vi "Main.vi"() -> ()   [LabVIEW 2013]
uses:
  Camera/lib/atmcd32d.llb/Shutter_type typedef.ctl
  Camera/lib/atmcd32d.llb/Shutter_mode typedef.ctl
  Utilities/controls/ctlSeqFNs_PI_SysNr.ctl
  Variables/StartStopMesaurement.vi
  Variables/GlobalExitVar.vi
  Variables/GlobalGetMesaurementStatus.vi
  Variables/GlobalSetGetConfigureCamera.vi
  Variables/ccdChipPixels.vi
  Variables/SavPath.vi
  Variables/GetPicture.vi
  Variables/StopGetPic.vi
  Variables/GlobalDevice.vi
  Variables/ScanrangeX.vi
  Variables/ScanrangeY.vi
  Variables/MesaurementModus.vi
  Variables/GlobalSetGetPixelOfRoi.vi
  Variables/GlobalSetConfigurationPhysikalInstruments.vi
  Variables/GlobalGetBeamDiagnostics.vi
  Variables/GlobalStopGetBeamDiagnostics.vi
panel:
  in  "Cams":enum32{"Acquisition", "Postprocessing"}(tab)
  out "Point":dbl[][](graph)
  out "Image Out":T1(plugin-control)
  in  "Gain::Value":dbl=16.0 min=16.0 max=64.0 step=1.0
  in  "Brightness::Value":dbl=127.0 min=0.0 max=254.0 step=1.0
  out "Image Number":u32
  out "Frame Rate":dbl
  in  "Stop Beam Diagnostic":bool
  in  "Get Beam Diagnostic":bool
  out "Final":dbl[][](graph)
  out "Confocal":dbl[][](graph)
  out "ISM":dbl[][](graph)
  in  "error in (no error)":errorcluster
  in  "Tab Control":enum32{"General"}(tab)
  in  "Check":bool
  in  "Stepsize Y":dbl format="%.2f"
  in  "Stepsize X":dbl format="%.2f"
  in  "Stepsize Z":dbl=10.0 format="%.2f"
  out "MesaurmentWarn":bool
  in  "Exposure (sec)":dbl=10.0 format="%.5f"
  in  "ModusMesaurement":enum32{"Fast", "Step"}(radio)
  in  "Scanrange Y":dbl format="%.2f"
  in  "Scanrange X":dbl format="%.2f"
  in  "Set Temp":bool
  in  "OpenShutter":bool
  in  "Emergency Exit":bool
  in  "Camera Settings":bool
  in  "GetPicture":bool
  in  "Stop Get Pic":bool
  in  "Close":bool
  in  "Start Measurement":bool
  in  "Move Mirror":bool
  in  "Move Scanner":bool
  in  "Set Workspace":bool
  in  "Laser Power":bool
  in  "AOTF Settings":bool
  in  "Device Choser":enum32{"Stage", "Mirror"}(radio)
  in  "Set CCD":bool
  in  "Startpoint X":dbl format="%.2f"
  in  "Startpoint Y":dbl format="%.2f"
  in  "Startpoint Z":dbl format="%.2f"
  in  "Scanrange Z":dbl=10.0 format="%.2f"
  in  "WAV":bool
  out "Writing":bool
  # "Data From Andor Camera Piped From Aquisition Process"
  # "Beam Diagnostic Camera"
  # "Beam Diagnostic Camera Controll"
  # "Define Where To Save the Mesaurement Data"
  # "Navigate In Sample Space & Choose Kinetic Device"
  # "Laser & AOTF/AOM"
  # "Data Acquisition Camera"
  # "Preview"
  # "Mesaurement Processs"
  # "Controlled & Emergency Shutdown"
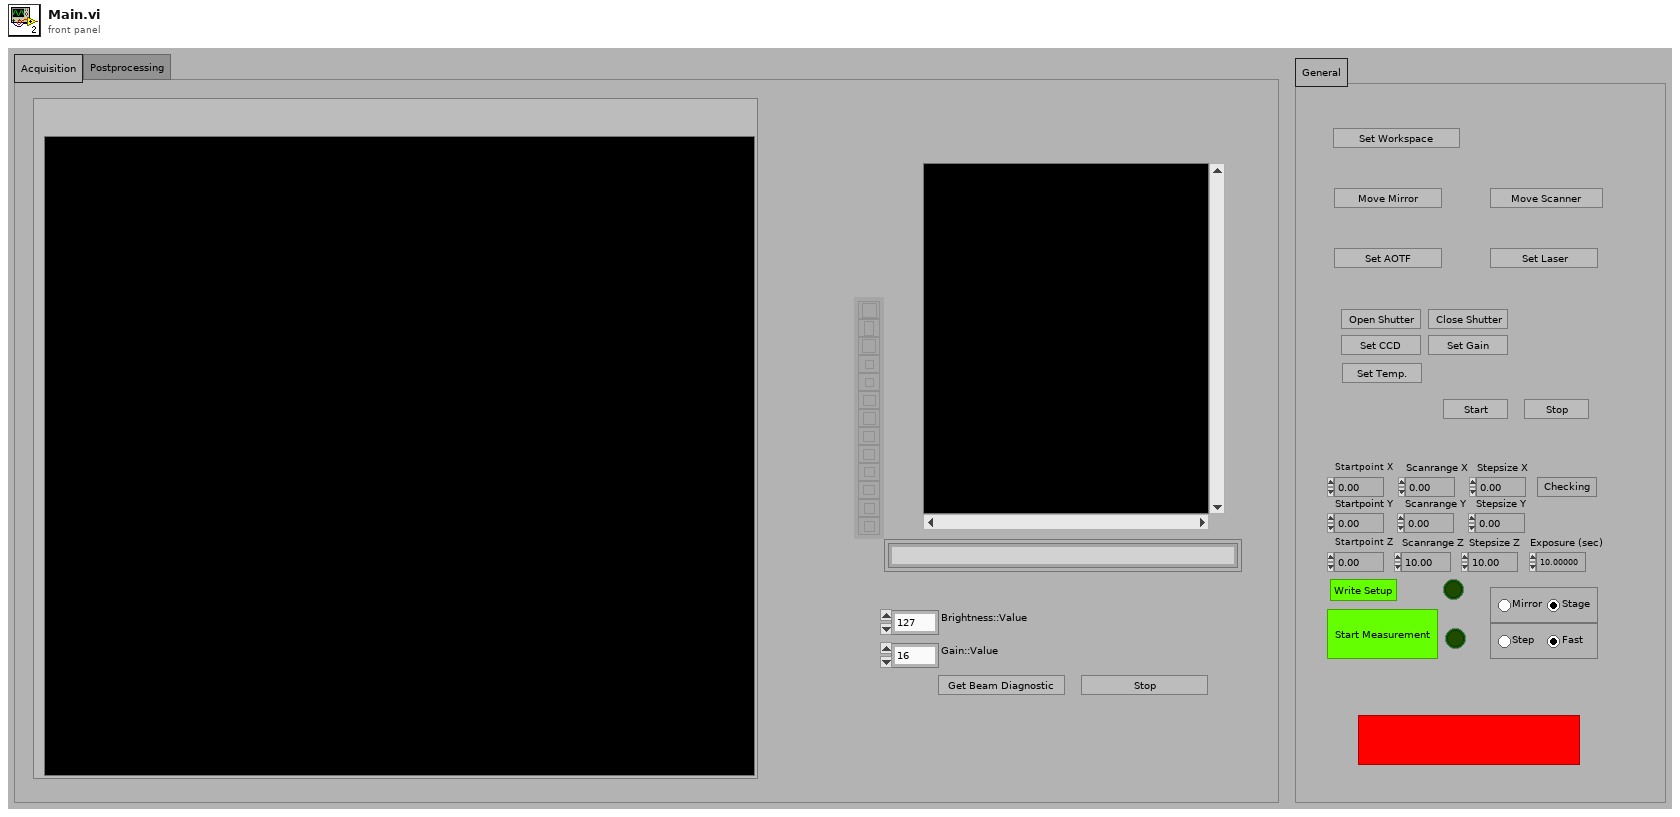
[diagram p1: front panel]
types:
  T1 = typedef "IMAQ Image.ctl" = refnum<image>
  T2 = typedef "Shutter_type typedef.ctl" = enum16{"TTL Low", "TTL High"}
  T3 = typedef "Shutter_mode typedef.ctl" = enum16{"Auto", "Open", "Close"}
  T4 = typedef "ctlSeqFNs_PI_SysNr.ctl" = enum16{"Zero", "E517", "E710"}
  T5 = cluster{"Conn. Axes scanner[0]":string, "Conn. Axes scanner[1]":string, "Conn. Axes scanner[2]":string}
  T6 = cluster{"Points":dbl, "J":dbl, "X length ":dbl, "J":dbl}
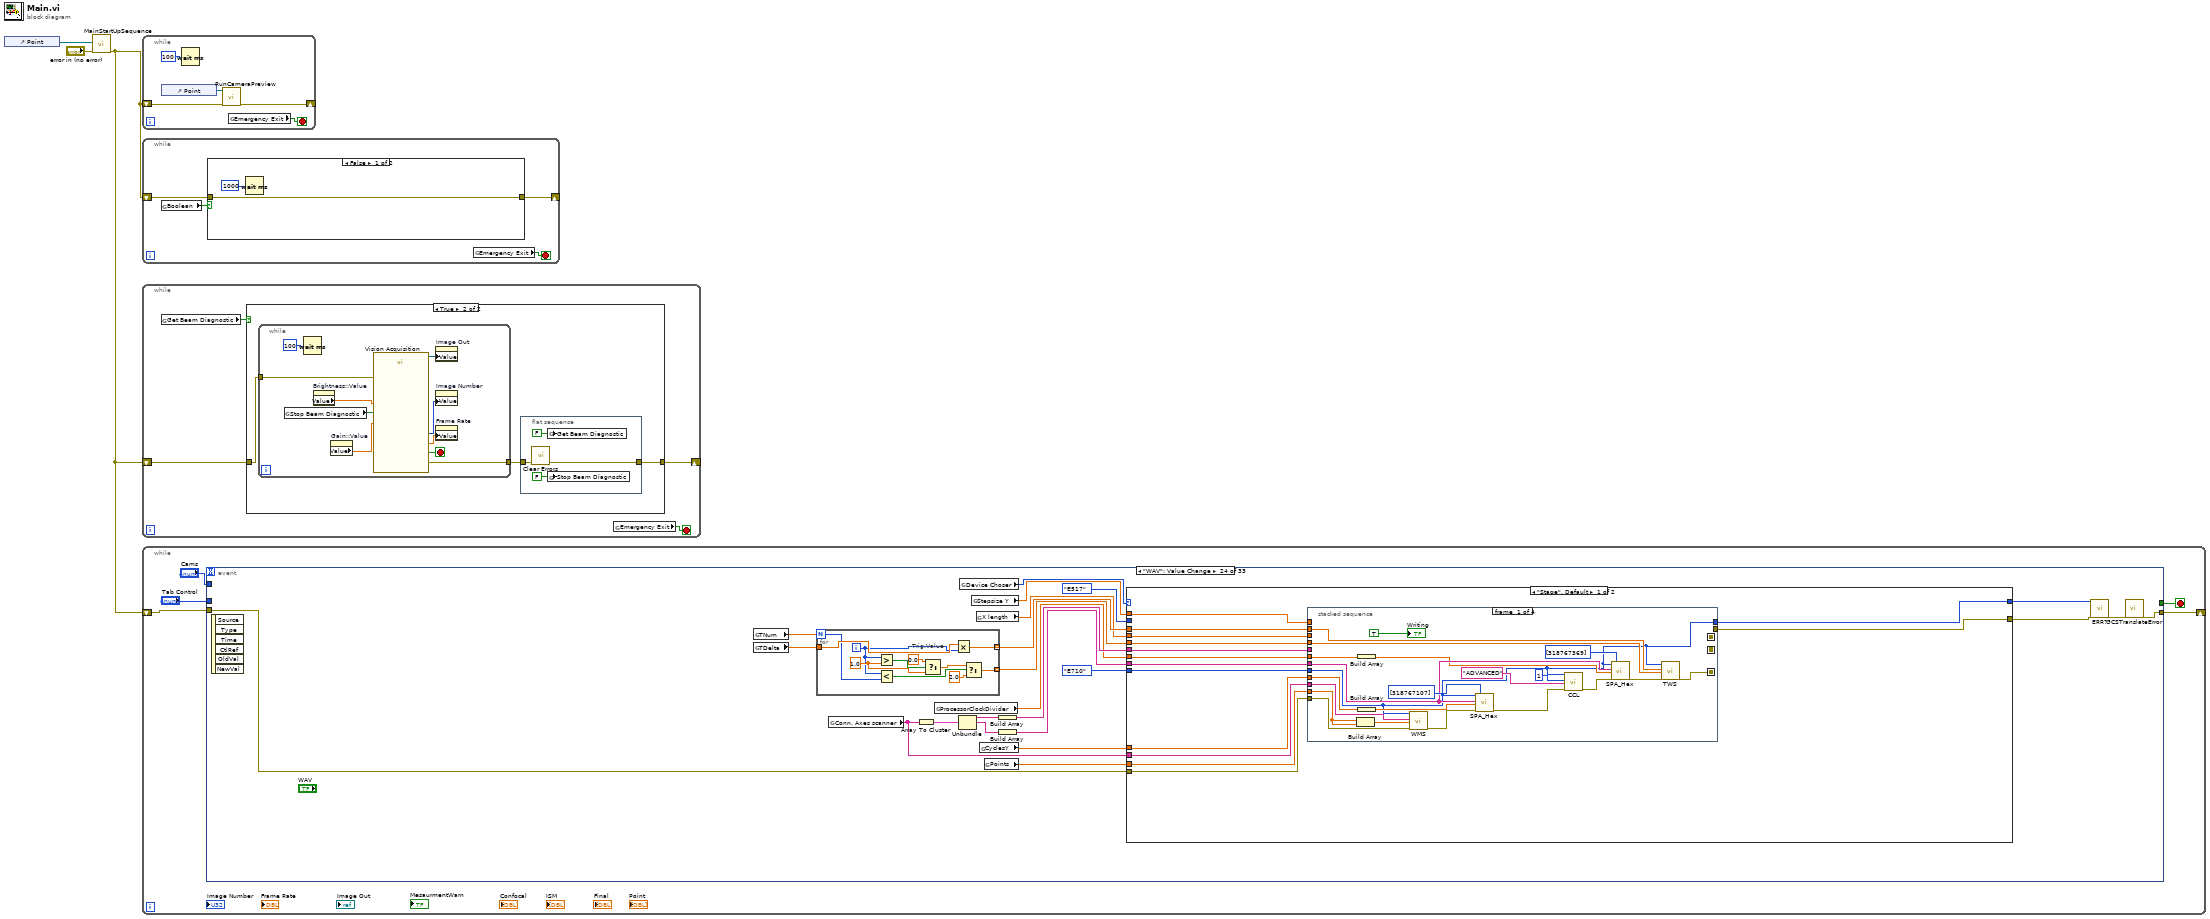
[diagram p0: block diagram]
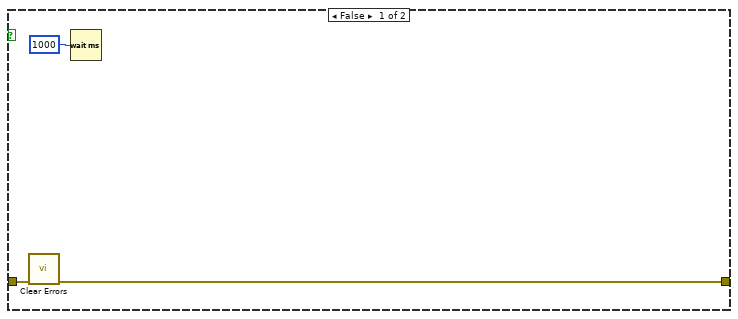
[diagram p2: hidden frame]
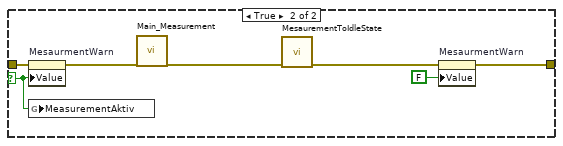
[diagram p3: hidden frame]
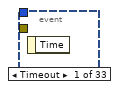
[diagram p4: hidden frame]
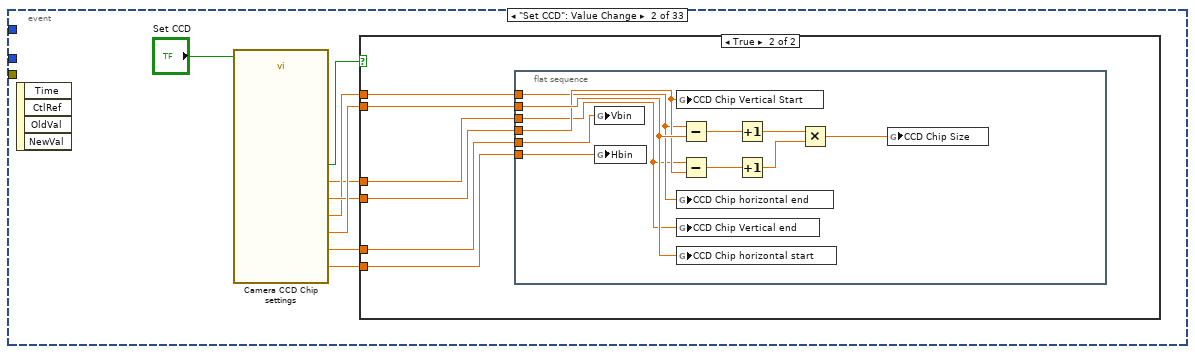
[diagram p5: hidden frame]
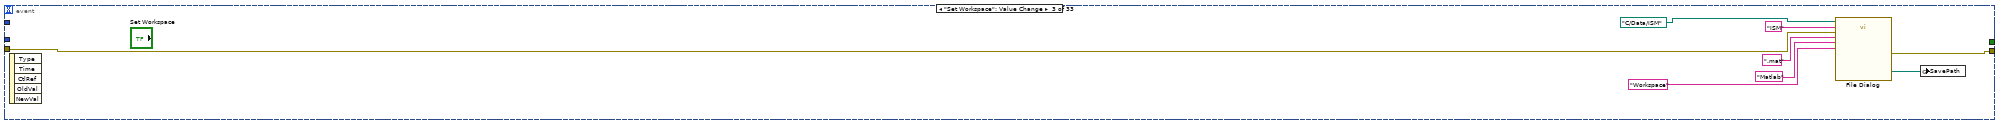
[diagram p7: hidden frame]
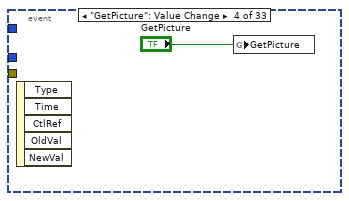
[diagram p8: hidden frame]
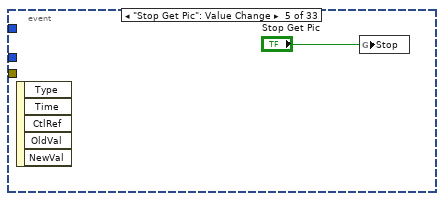
[diagram p9: hidden frame]
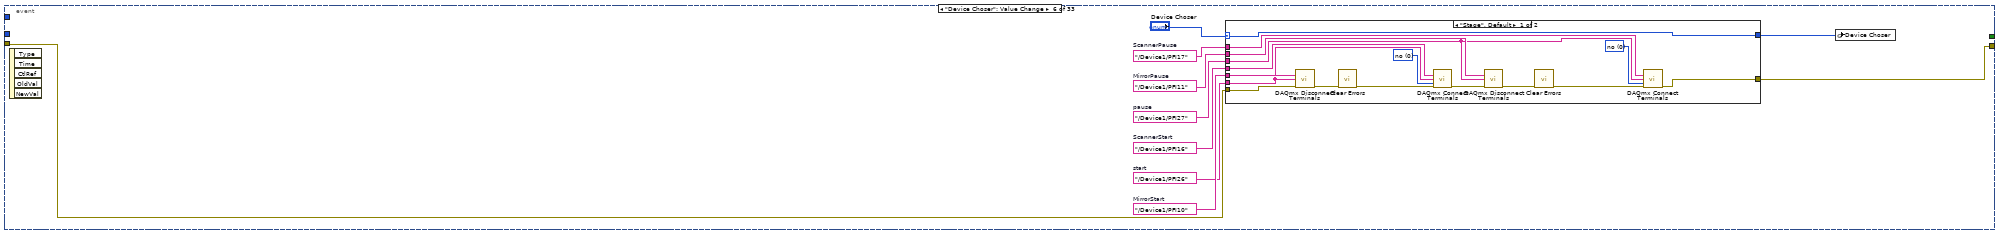
[diagram p10: hidden frame]
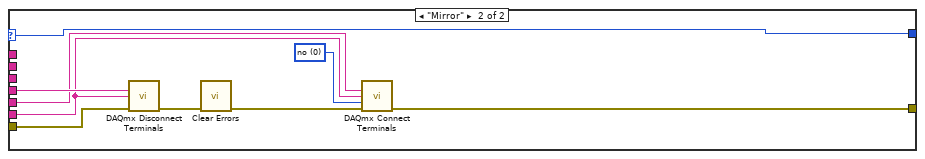
[diagram p11: hidden frame]
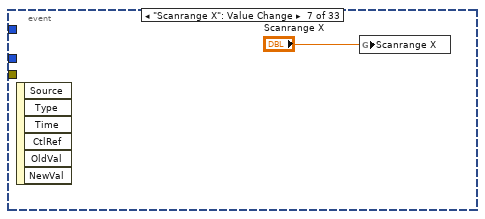
[diagram p12: hidden frame]
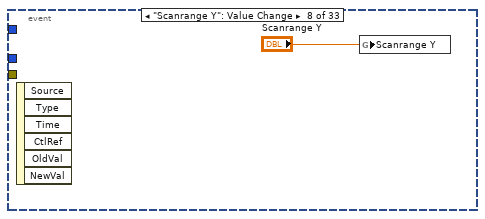
[diagram p13: hidden frame]
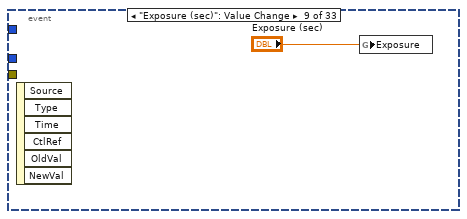
[diagram p14: hidden frame]
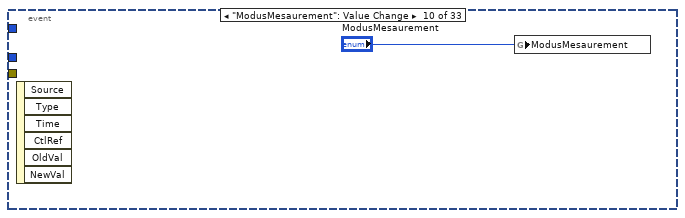
[diagram p15: hidden frame]
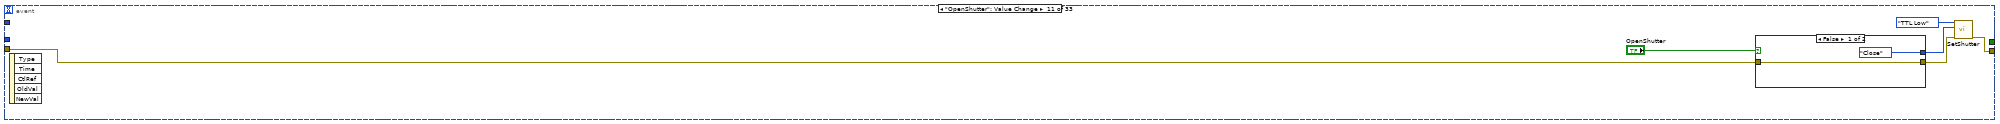
[diagram p16: hidden frame]
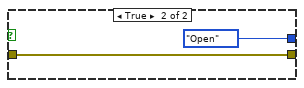
[diagram p17: hidden frame]
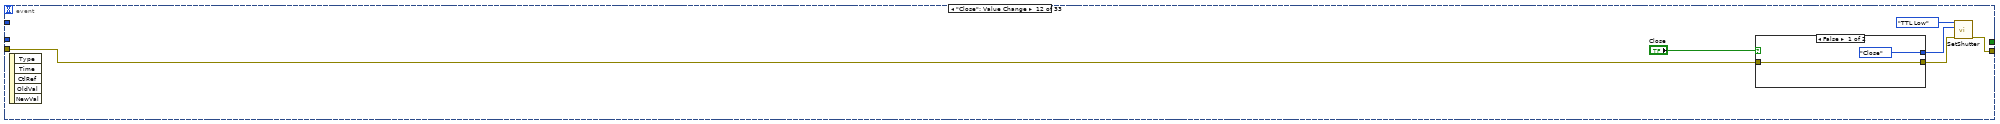
[diagram p18: hidden frame]
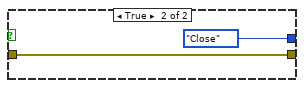
[diagram p19: hidden frame]
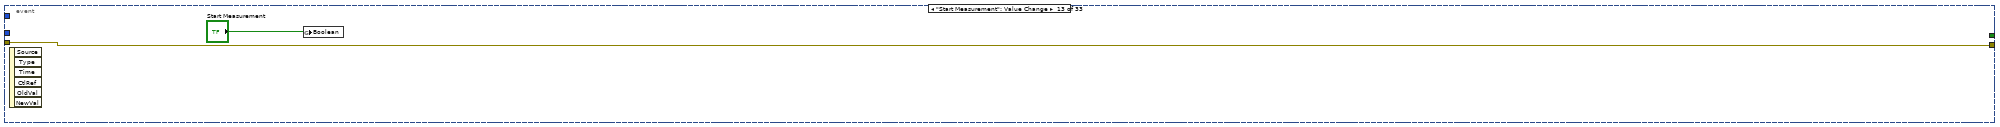
[diagram p20: hidden frame]
diagram:
  n1 = control-ref of="Point"() -> (w1:refnum<vi>)
  n2 = call "MainStartUpSequence.vi"("IntGraph Refnum"=w1, "error in (no error)"="error in (no error)") -> ("error out"=w2:errorcluster)  [unwired: 15 in, 2 out]
  n3 = while {
    shift-right: [w6] -> _
    shift-left: w2 -> [w7]
    stop <- w8 stop-if-true
    n4 = control-ref of="Point"() -> (w5:refnum<vi>)
    n5 = Wait (ms)(milliseconds to wait=u32 100) -> ()  [unwired: 1 out]
    n6 = call "RunCameraPreview.vi"("error in (no error)"=w7, "IntensityGraph in"=w5) -> ("error out"=w6:errorcluster)  [unwired: 9 in]
    n7 = global read "GlobalExitVar.vi" "Emergency Exit"() -> (w8:bool)
  }
  n8 = while {
    shift-right: [w11] -> _
    shift-left: w2 -> [w12]
    stop <- w9 stop-if-true
    n9 = global read "StartStopMesaurement.vi" "Boolean"() -> (w10:bool)
    n10 = case shown="False" w10 {
      selector: w10 -> [_ w15]
      tunnel: w12 -> [w13 w17]
      tunnel: [w13 w19] -> w11
      frame False {
        n11 = Wait (ms)(milliseconds to wait=u32 1000) -> ()  [unwired: 1 out]
      }
      frame True {
        n12 = property on="MesaurmentWarn" class="Bool (strict)"(error in=w17, "Value"=w15) -> (error out=w16:errorcluster)  [unwired: 1 in, 1 out]
        n13 = global write "GlobalGetMesaurementStatus.vi" "MeasurementAktiv"(w15) -> ()
        n14 = call "Main_Measurement.vi"("error in"=w16) -> ("error out"=w21:errorcluster)  [unwired: 18 in]
        n15 = call "MesaurementToIdleState.vi"("error in (no error)"=w21) -> ("error out"=w20:errorcluster)  [unwired: 10 in]
        n16 = property on="MesaurmentWarn" class="Bool (strict)"(error in=w20, "Value"=FALSE ("MesaurmentWarn")) -> (error out=w19:errorcluster)  [unwired: 1 in, 1 out]
      }
    }
    n17 = global read "GlobalExitVar.vi" "Emergency Exit"() -> (w9:bool)
  }
  n18 = while {
    shift-right: [w23] -> _
    shift-left: w2 -> [w24]
    stop <- w25 stop-if-true
    n19 = global read "GlobalGetBeamDiagnostics.vi" "Get Beam Diagnostic"() -> (w22:bool)
    n20 = case shown="True" w22 {
      tunnel: w24 -> [w27 w31]
      tunnel: [w26 w30] -> w23
      frame False {
        n21 = call <vilib>:"Clear Errors.vi"("error in (no error)"=w27) -> ("error out"=w26:errorcluster)  [unwired: 6 in]
        n22 = Wait (ms)(milliseconds to wait=u32 1000) -> ()  [unwired: 1 out]
      }
      frame True {
        n23 = while {
          tunnel: w31 -> [w40]
          tunnel: [w39] -> w29
          stop <- w41 stop-if-true
          n24 = global read "GlobalStopGetBeamDiagnostics.vi" "Stop Beam Diagnostic"() -> (w38:bool)
          n25 = Wait (ms)(milliseconds to wait=u32 100) -> ()  [unwired: 1 out]
          n26 = property on="Brightness::Value" class="DigNum (strict)"() -> ("Value"=w37:dbl)  [unwired: 2 in, 2 out]
          n27 = property on="Gain::Value" class="DigNum (strict)"() -> ("Value"=w36:dbl)  [unwired: 2 in, 2 out]
          n28 = call "Vision Acquisition"("Brightness::Value"=w37, "Stop (F)"=w38, "Gain::Value"=w36, "error in"=w40) -> ("Image Out"=w33:T1, "Image Number"=w35:u32, "Frame Rate"=w34:dbl, "Stopped"=w41:bool, "error out"=w39:errorcluster)  [unwired: 19 in]
          n29 = property on="Image Out" class="ImageControl"("Value"=w33) -> ()  [unwired: 2 in, 2 out]
          n30 = property on="Image Number" class="DigNum (strict)"("Value"=w35) -> ()  [unwired: 2 in, 2 out]
          n31 = property on="Frame Rate" class="DigNum (strict)"("Value"=w34) -> ()  [unwired: 2 in, 2 out]
        }
        n32 = flat-sequence {
          tunnel: [w42] -> w30
          tunnel: w29 -> [w43]
          frame #0 {
            n33 = call <vilib>:"Clear Errors.vi"("error in (no error)"=w43) -> ("error out"=w42:errorcluster)  [unwired: 6 in]
            n34 = global write "GlobalGetBeamDiagnostics.vi" "Get Beam Diagnostic"(FALSE ("Get Beam Diagnostic")) -> ()
            n35 = global write "GlobalStopGetBeamDiagnostics.vi" "Stop Beam Diagnostic"(FALSE ("Stop Beam Diagnostic")) -> ()
          }
        }
      }
    }
    n36 = global read "GlobalExitVar.vi" "Emergency Exit"() -> (w25:bool)
  }
  n37 = while "User Events" {
    shift-right: [w48] -> _
    shift-left: w2 -> [w50]
    stop <- w49 stop-if-true
    n38 = event shown="[23] \"WAV\": Value Change" {
      selector: _ -> [_ _ _ _ _ _ _ _ _ _ _ _ _ _ _ _ _ _ _ _ _ _ _ _ _ _ _ _ _ _ _ _ _]
      dyn-events: _ -> [_ _ _ _ _ _ _ _ _ _ _ _ _ _ _ _ _ _ _ _ _ _ _ _ _ _ _ _ _ _ _ _ _]
      timeout: _ -> [_ _ _ _ _ _ _ _ _ _ _ _ _ _ _ _ _ _ _ _ _ _ _ _ _ _ _ _ _ _ _ _ _]
      tunnel: [_ _ w77 _ _ w90 _ _ _ _ w126 w136 w146 w148 w161 w179 _ _ _ _ _ _ _ w281 _ w431 _ _ w495 w496 _ _ w502] -> w48
      tunnel: w50 -> [_ _ w76 _ _ w91 _ _ _ _ w128 w138 w146 w153 w165 w183 _ _ _ _ _ _ _ w276 w400 w422 _ _ w494 w497 _ _ w506]
      tunnel: [_ _ _ _ _ _ _ _ _ _ _ _ _ _ _ _ _ _ _ _ _ _ _ _ _ _ _ _ _ _ _ _ w501] -> w49
      tunnel: "Tab Control" -> [_ _ _ _ _ _ _ _ _ _ _ _ _ _ _ _ _ _ _ _ _ _ _ _ _ _ _ _ _ _ _ _ _]
      tunnel: "Cams" -> [_ _ _ _ _ _ _ _ _ _ _ _ _ _ _ _ _ _ _ _ _ _ _ _ _ _ _ _ _ _ _ _ _]
      event Timeout {
        n39 = event-data() -> ()  [unwired: 1 in, 1 out]
      }
      event "Set CCD": Value Change {
        n40 = event-data() -> ()  [unwired: 1 in, 4 out]
        n41 = call "Camera CCD Chip settings"("Enable"="Set CCD") -> ("Horizontal Binning"=w51:dbl, "Vertical Binning"=w56:dbl, "CCD Chip Horizontal Start"=w55:dbl, "CCD Chip Horizontal End"=w53:dbl, "CCD Chip Vertical Start"=w54:dbl, "CCD Chip Vertical End"=w52:dbl, "OK"=w57:bool)  [unwired: 11 in, 1 out]
        n42 = case shown="True" w57 {
          tunnel: w56 -> [_ w64]
          tunnel: w55 -> [_ w63]
          tunnel: w54 -> [_ w62]
          tunnel: w53 -> [_ w61]
          tunnel: w52 -> [_ w60]
          tunnel: w51 -> [_ w59]
          frame False {
          }
          frame True {
            n43 = flat-sequence {
              tunnel: w64 -> [w70]
              tunnel: w63 -> [w69]
              tunnel: w62 -> [w68]
              tunnel: w61 -> [w67]
              tunnel: w60 -> [w66]
              tunnel: w59 -> [w65]
              frame #0 {
                n44 = global write "GlobalSetGetConfigureCamera.vi" "Vbin"(w70) -> ()
                n45 = global write "GlobalSetGetConfigureCamera.vi" "Hbin"(w65) -> ()
                n46 = global write "ccdChipPixels.vi" "CCD Chip Vertical Start"(w68) -> ()
                n47 = global write "ccdChipPixels.vi" "CCD Chip horizontal end"(w67) -> ()
                n48 = global write "ccdChipPixels.vi" "CCD Chip Vertical end"(w66) -> ()
                n49 = global write "ccdChipPixels.vi" "CCD Chip horizontal start"(w69) -> ()
                n50 = Subtract(x=w67, y=w69) -> (x-y=w72:dbl)
                n51 = Subtract(x=w66, y=w68) -> (x-y=w71:dbl)
                n52 = Increment(x=w72) -> (x+1=w74:dbl)
                n53 = Increment(x=w71) -> (x+1=w73:dbl)
                n54 = Multiply(x=w74, y=w73) -> (x*y=w75:dbl)
                n55 = global write "ccdChipPixels.vi" "CCD Chip Size"(w75) -> ()
              }
            }
          }
        }
      }
      event "Set Workspace": Value Change {
        n56 = event-data() -> ()  [unwired: 1 in, 5 out]
        n57 = call "File Dialog"("start path"=path "C:/Data/ISM", "button label"="Workspace", "default name"="ISM", "error in"=w76, "pattern (all files)"=".mat", "pattern label"="Matlab") -> ("selected path"=w82:path, "error out"=w77:errorcluster)  [unwired: 6 in, 2 out]
        n58 = global write "SavPath.vi" "SavePath"(w82) -> ()
      }
      event "GetPicture": Value Change {
        n59 = event-data() -> ()  [unwired: 1 in, 5 out]
        n60 = global write "GetPicture.vi" "GetPicture"("GetPicture") -> ()
      }
      event "Stop Get Pic": Value Change {
        n61 = event-data() -> ()  [unwired: 1 in, 5 out]
        n62 = global write "StopGetPic.vi" "Stop"("Stop Get Pic") -> ()
      }
      event "Device Choser": Value Change {
        w87 = tag "/Device1/PFI17"  # ScannerPause
        w88 = tag "/Device1/PFI11"  # MirrorPause
        w86 = tag "/Device1/PFI26"  # start
        w89 = tag "/Device1/PFI27"  # pause
        w95 = tag "/Device1/PFI16"  # ScannerStart
        w94 = tag "/Device1/PFI10"  # MirrorStart
        n63 = event-data() -> ()  [unwired: 1 in, 5 out]
        n64 = case shown="\"Stage\", Default" "Device Choser" {
          selector: "Device Choser" -> [w104 w112]
          tunnel: w91 -> [w110 w118]
          tunnel: [w96 w120] -> w90
          tunnel: w94 -> [w108 w113]
          tunnel: w86 -> [w107 w116]
          tunnel: w95 -> [w109 w117]
          tunnel: [w104 w112] -> w92
          tunnel: w89 -> [w98 _]
          tunnel: w88 -> [w100 _]
          tunnel: w87 -> [w99 _]
          frame "Stage", Default {
            w103 = 0 items=["no", "yes"] ("invert polarity")
            w111 = 0 items=["no", "yes"] ("invert polarity")
            n65 = call <vilib>:"DAQmx Disconnect Terminals.vi"("source terminal"=w108, "destination terminal"=w107, "error in"=w110) -> ("error out"=w106:errorcluster)  [unwired: 12 in]
            n66 = call <vilib>:"Clear Errors.vi"("error in (no error)"=w106) -> ("error out"=w105:errorcluster)  [unwired: 6 in]
            n67 = call <vilib>:"DAQmx Connect Terminals.vi"("source terminal"=w109, "destination terminal"=w107, "invert polarity"=w111, "error in"=w105) -> ("error out"=w97:errorcluster)  [unwired: 11 in]
            n68 = call <vilib>:"DAQmx Disconnect Terminals.vi"("source terminal"=w100, "destination terminal"=w98, "error in"=w97) -> ("error out"=w102:errorcluster)  [unwired: 12 in]
            n69 = call <vilib>:"Clear Errors.vi"("error in (no error)"=w102) -> ("error out"=w101:errorcluster)  [unwired: 6 in]
            n70 = call <vilib>:"DAQmx Connect Terminals.vi"("source terminal"=w99, "destination terminal"=w98, "invert polarity"=w103, "error in"=w101) -> ("error out"=w96:errorcluster)  [unwired: 11 in]
          }
          frame "Mirror" {
            w119 = 0 items=["no", "yes"] ("invert polarity")
            n71 = call <vilib>:"DAQmx Disconnect Terminals.vi"("source terminal"=w117, "destination terminal"=w116, "error in"=w118) -> ("error out"=w115:errorcluster)  [unwired: 12 in]
            n72 = call <vilib>:"Clear Errors.vi"("error in (no error)"=w115) -> ("error out"=w114:errorcluster)  [unwired: 6 in]
            n73 = call <vilib>:"DAQmx Connect Terminals.vi"("source terminal"=w113, "destination terminal"=w116, "invert polarity"=w119, "error in"=w114) -> ("error out"=w120:errorcluster)  [unwired: 11 in]
          }
        }
        n74 = global write "GlobalDevice.vi" "Device Choser"(w92) -> ()
      }
      event "Scanrange X": Value Change {
        n75 = event-data() -> ()  [unwired: 1 in, 6 out]
        n76 = global write "ScanrangeX.vi" "Scanrange X"("Scanrange X") -> ()
      }
      event "Scanrange Y": Value Change {
        n77 = event-data() -> ()  [unwired: 1 in, 6 out]
        n78 = global write "ScanrangeY.vi" "Scanrange Y"("Scanrange Y") -> ()
      }
      event "Exposure (sec)": Value Change {
        n79 = event-data() -> ()  [unwired: 1 in, 6 out]
        n80 = global write "GlobalSetGetConfigureCamera.vi" "Exposure"("Exposure (sec)") -> ()
      }
      event "ModusMesaurement": Value Change {
        n81 = event-data() -> ()  [unwired: 1 in, 6 out]
        n82 = global write "MesaurementModus.vi" "ModusMesaurement"("ModusMesaurement") -> ()
      }
      event "OpenShutter": Value Change {
        n83 = event-data() -> ()  [unwired: 1 in, 5 out]
        n84 = case shown="False" "OpenShutter" {
          tunnel: [Shutter_mode_typedef."Close" ("mode") Shutter_mode_typedef."Open" ("mode")] -> w130
          tunnel: w128 -> [w132 w133]
          tunnel: [w132 w133] -> w127
          frame False {
          }
          frame True {
          }
        }
        n85 = call "SetShutter.vi"("type"=Shutter_type_typedef."TTL Low", "mode"=w130, "error in (no error)"=w127) -> ("error out"=w126:errorcluster)  [unwired: 11 in, 1 out]
      }
      event "Close": Value Change {
        n86 = event-data() -> ()  [unwired: 1 in, 5 out]
        n87 = case shown="False" "Close" {
          tunnel: w138 -> [w141 w144]
          tunnel: [w141 w144] -> w137
          tunnel: [Shutter_mode_typedef."Close" ("mode") Shutter_mode_typedef."Close" ("mode")] -> w135
          frame False {
          }
          frame True {
          }
        }
        n88 = call "SetShutter.vi"("type"=Shutter_type_typedef."TTL Low", "mode"=w135, "error in (no error)"=w137) -> ("error out"=w136:errorcluster)  [unwired: 11 in, 1 out]
      }
      event "Start Measurement": Value Change {
        n89 = event-data() -> ()  [unwired: 1 in, 6 out]
        n90 = global write "StartStopMesaurement.vi" "Boolean"("Start Measurement") -> ()
      }
      event "Move Scanner": Value Change {
        n91 = event-data() -> ()  [unwired: 1 in, 6 out]
        n92 = call "Scanner kinetics"("error in (no error)"=w153) -> ("Go to Z-position"=w150:dbl, "Go to Y-position"=w151:dbl, "Go to X-position"=w152:dbl, "OK"=w149:bool, "error out"=w147:errorcluster)  [unwired: 14 in]
        n93 = case shown="True" w149 {
          tunnel: w152 -> [_ w159]
          tunnel: w151 -> [_ w158]
          tunnel: w150 -> [_ w157]
          tunnel: [w154 w156] -> w148
          tunnel: w147 -> [w154 w155]
          frame False {
          }
          frame True {
            n94 = call "Scanner_Mirror_configuration.vi"("POS X"=w159, "POS Y"=w158, "POS Z"=w157, "error in"=w155) -> ("error out"=w156:errorcluster)  [unwired: 15 in]
          }
        }
      }
      event "Move Mirror": Value Change {
        n95 = event-data() -> ()  [unwired: 1 in, 6 out]
        n96 = call "Mirror kinetics"("error in (no error)"=w165) -> ("Go to X-position"=w163:dbl, "Go to Y-position"=w164:dbl, "OK"=w160:bool, "error out"=w162:errorcluster)  [unwired: 15 in]
        n97 = case shown="True" w160 {
          tunnel: w164 -> [_ w170]
          tunnel: w163 -> [_ w169]
          tunnel: w162 -> [w166 w168]
          tunnel: [w166 w167] -> w161
          frame False {
          }
          frame True {
            n98 = call "MoveMirror.vi"("error in 2"=w168, "POS X rad"=w169, "POS Y rad"=w170) -> ("error out 2"=w167:errorcluster)  [unwired: 1 in]
          }
        }
      }
      event "Check": Value Change {
        n99 = event-data() -> ()  [unwired: 1 in, 6 out]
        n100 = global read "ScanrangeX.vi" "Scanrange X"() -> (w178:dbl)
        n101 = global read "ScanrangeY.vi" "Scanrange Y"() -> (w177:dbl)
        n102 = global read "GlobalSetGetPixelOfRoi.vi" "Stepsize Y"() -> (w188:dbl)
        n103 = global read "GlobalSetGetPixelOfRoi.vi" "Stepsize X"() -> (w191:dbl)
        n104 = global write "GlobalSetGetPixelOfRoi.vi" "X length"(w178) -> ()
        n105 = global write "GlobalSetGetPixelOfRoi.vi" "Y length"(w177) -> ()
        n106 = Quotient & Remainder(x=w178, y=w191) -> (x-y*floor(x/y)=w190:dbl)  [unwired: 1 out]
        n107 = Quotient & Remainder(x=w177, y=w188) -> (x-y*floor(x/y)=w189:dbl)  [unwired: 1 out]
        n108 = Greater Than 0?(x=w190) -> (x > 0?=w187:bool)
        n109 = Greater Than 0?(x=w189) -> (x > 0?=w186:bool)
        n110 = Or(x=w187, y=w186) -> (x .or. y?=w185:bool)
        n111 = case shown="True" w185 {
          tunnel: w183 -> [w232 w234]
          tunnel: [w232 w233] -> w180
          frame False {
          }
          frame True {
            n112 = call "Display Message to User3"("error in (no error)"=w234) -> ("error out"=w233:errorcluster)  [unwired: 9 in, 1 out]
          }
        }
        n113 = global read "GlobalSetGetConfigureCamera.vi" "Exposure"() -> (w171:sgl)
        n114 = global read "GlobalDevice.vi" "Device Choser"() -> (w198:enum32{"Stage", "Mirror"})
        n115 = global read "GlobalSetGetPixelOfRoi.vi" "Stack length"() -> (w192:dbl)
        n116 = case shown="\"Stage\", Default" w198 {
          tunnel: [w244 w255] -> w211
          tunnel: [w239 w251] -> w194
          tunnel: [w245 w256] -> w204
          tunnel: [w241 w250] -> w199
          tunnel: [w243 w254] -> w197
          tunnel: w178 -> [w245 w256]
          tunnel: w177 -> [w244 w255]
          tunnel: w188 -> [w243 w254]
          tunnel: w191 -> [w241 w250]
          tunnel: w171 -> [w240 w249]
          tunnel: [w238 w253] -> w193
          tunnel: w192 -> [w238 w253]
          tunnel: [w237 w248] -> w181
          tunnel: w180 -> [w237 w248]
          tunnel: [5000.0 ("input variable") 25000.0 ("input variable")] -> w173
          tunnel: [63488.0 ("input variable") 63488.0 ("input variable")] -> w174
          frame "Stage", Default {
            n117 = Divide(x=w241, y=w240) -> (x/y=w242:dbl)
            n118 = Round To Nearest(number=w242) -> (nearest integer value=w239:dbl)
          }
          frame "Mirror" {
            # "1 durch25000 fehlt speed calc \nbei spiegel anpassen dh 8.2.14"
            n119 = Divide(x=w250, y=w249) -> (x/y=w252:dbl)
            n120 = Round To Nearest(number=w252) -> (nearest integer value=w251:dbl)
          }
        }
        n121 = global read "GlobalSetGetPixelOfRoi.vi" "Stepsize Z"() -> (w196:dbl)
        n122 = while {
          tunnel: w211 -> [w231]
          tunnel: [w219] -> w210
          tunnel: [w230] -> w209
          tunnel: [w229] -> w208
          tunnel: [w228] -> w207
          tunnel: w204 -> [w227]
          tunnel: w199 -> [w226]
          tunnel: w197 -> [w225]
          tunnel: w196 -> [w224]
          tunnel: w194 -> [w218]
          tunnel: w193 -> [w223]
          tunnel: [w222] -> w184
          tunnel: [w221] -> w176
          tunnel: w174 -> [w220]
          shift-right: [w215] -> _
          shift-left: _ -> [w216]
          tunnel: w173 -> [w214]
          tunnel: [w213] -> w172
          i -> [w213]
          stop <- w217 stop-if-true
          n123 = formula code="CyclesY = floor (RangeY/StepY) + 1;\nCyclesZ = floor (RangeZ/StepZ) + 1;\nVmin = Clock/Memory * RangeX * (1 + CyclesY);\nPointsX = RangeX / Speed * 10000;\nTDelta = PointsX / RangeX * Trigger;\nTNum = floor ( PointsX / TDelta);"("RangeX"=w227, "RangeY"=w231, "RangeZ"=w223, "StepY"=w225, "StepZ"=w224, "Speed"=w218, "Trigger"=w226, "Clock"=w216, "Memory"=w220) -> ("Vmin"=w219:dbl, "CyclesY"=w221:dbl, "CyclesZ"=w228:dbl, "PointsX"=w222:dbl, "TDelta"=w230:dbl, "TNum"=w229:dbl)
          n124 = Greater?(x=w218, y=w219) -> (0:w217:bool)
          n125 = Divide(x=w214, y=w213) -> (x/y=w215:dbl)
        }
        n126 = global write "GlobalSetGetPixelOfRoi.vi" "Stepsize Y"(w197) -> ()
        n127 = global write "GlobalSetGetPixelOfRoi.vi" "Points"(w184) -> ()
        n128 = global write "GlobalSetGetPixelOfRoi.vi" "TDelta"(w209) -> ()
        n129 = global write "GlobalDevice.vi" "ProcessorClockDivider"(w172) -> ()
        n130 = global write "GlobalSetGetPixelOfRoi.vi" "TNum"(w208) -> ()
        n131 = global write "GlobalSetGetPixelOfRoi.vi" "CyclesY"(w176) -> ()
        n132 = global write "GlobalSetGetPixelOfRoi.vi" "CyclesZ"(w207) -> ()
        n133 = Less?(x=w194, y=w210) -> (x < y?=w212:bool)
        n134 = Divide(x=w204, y=w199) -> (x/y=w175:dbl)
        n135 = Subtract(x=w176, y=1.0) -> (x-y=w200:dbl)
        n136 = Multiply(x=w200, y=w175) -> (x*y=w206:dbl)
        n137 = Multiply(x=50.0, y=w176) -> (x*y=w202:dbl)
        n138 = case shown="\"Stage\", Default" w198 {
          tunnel: w206 -> [w258 _]
          tunnel: [w258 w260] -> w205
          tunnel: w202 -> [_ w260]
          tunnel: [w257 w259] -> w182
          tunnel: w181 -> [w257 w259]
          frame "Stage", Default {
          }
          frame "Mirror" {
          }
        }
        n139 = global write "GlobalSetGetConfigureCamera.vi" "Kinetics"(w205) -> ()
        n140 = case shown="False" w212 {
          tunnel: w210 -> [_ w265]
          tunnel: [w263 w265] -> w195
          tunnel: w194 -> [w263 _]
          tunnel: w182 -> [w262 w264]
          tunnel: [w261 w264] -> w179
          frame False {
            n141 = call "Display Message to User2"("error in (no error)"=w262) -> ("error out"=w261:errorcluster)  [unwired: 9 in, 1 out]
          }
          frame True {
            n142 = call "Display Message to User"() -> ()  [unwired: 10 in, 2 out]
          }
        }
        n143 = global write "GlobalSetGetPixelOfRoi.vi" "Scanspeed"(w195) -> ()
      }
      event "Scanrange Z": Value Change {
        n144 = event-data() -> ()  [unwired: 1 in, 6 out]
        n145 = global write "GlobalSetGetPixelOfRoi.vi" "Stack length"("Scanrange Z") -> ()
      }
      event "Startpoint X": Value Change {
        n146 = event-data() -> ()  [unwired: 1 in, 6 out]
        n147 = global write "GlobalSetGetPixelOfRoi.vi" "X Start"("Startpoint X") -> ()
      }
      event "Startpoint Y": Value Change {
        n148 = event-data() -> ()  [unwired: 1 in, 6 out]
        n149 = global write "GlobalSetGetPixelOfRoi.vi" "Y Start"("Startpoint Y") -> ()
      }
      event "Startpoint Z": Value Change {
        n150 = event-data() -> ()  [unwired: 1 in, 6 out]
        n151 = global write "GlobalSetGetPixelOfRoi.vi" "Stack Start"("Startpoint Z") -> ()
      }
      event "Stepsize Z": Value Change {
        n152 = event-data() -> ()  [unwired: 1 in, 6 out]
        n153 = global write "GlobalSetGetPixelOfRoi.vi" "Stepsize Z"("Stepsize Z") -> ()
      }
      event "Stepsize X": Value Change {
        n154 = event-data() -> ()  [unwired: 1 in, 6 out]
        n155 = global write "GlobalSetGetPixelOfRoi.vi" "Stepsize X"("Stepsize X") -> ()
      }
      event "Stepsize Y": Value Change {
        n156 = event-data() -> ()  [unwired: 1 in, 6 out]
        n157 = global write "GlobalSetGetPixelOfRoi.vi" "Stepsize Y"("Stepsize Y") -> ()
      }
      event "WAV": Value Change {
        n158 = event-data() -> ()  [unwired: 1 in, 6 out]
        n159 = global read "GlobalSetGetPixelOfRoi.vi" "TNum"() -> (w273:dbl)
        n160 = global read "GlobalSetGetPixelOfRoi.vi" "TDelta"() -> (w274:dbl)
        n161 = for {
          N: w273 -> [w391]
          tunnel: w274 -> [w397]
          tunnel: [w396] -> w288 mode=indexing
          tunnel: [w387] -> w287 mode=indexing
          i -> [w392]
          w394 = 1.0 ("f")
          # "Trig.Value"
          n162 = Greater?(x=w392, y=w394) -> (0:w393:bool)
          n163 = Less?(x=w392, y=w391) -> (x < y?=w390:bool)
          n164 = Select(t=0.0 ("f"), s=w393, f=w394) -> (s? t:f=w389:dbl)
          n165 = Multiply(x=w397, y=w392) -> (x*y=w396:dbl)
          n166 = Select(t=w389, s=w390, f=2.0) -> (s? t:f=w387:dbl)
        }
        n167 = global read "GlobalSetConfigurationPhysikalInstruments.vi" "Conn. Axes scanner"() -> (w295:string[])
        n168 = Array To Cluster(array=w295) -> (cluster=w289:T5)
        n169 = global read "GlobalDevice.vi" "ProcessorClockDivider"() -> (w275:dbl)
        n170 = Unbundle(w289) -> ("Conn. Axes scanner[0]"=w291:string, "Conn. Axes scanner[1]"=w290:string)  [unwired: 1 out]
        n171 = global read "GlobalDevice.vi" "Device Choser"() -> (w278:enum32{"Stage", "Mirror"})
        n172 = global read "GlobalSetGetPixelOfRoi.vi" "Stepsize Y"() -> (w286:dbl)
        n173 = global read "GlobalSetGetPixelOfRoi.vi" "X length"() -> (w285:dbl)
        n174 = global read "GlobalSetGetPixelOfRoi.vi" "CyclesY"() -> (w284:dbl)
        n175 = global read "GlobalSetGetPixelOfRoi.vi" "Points"() -> (w283:dbl)
        n176 = Build Array(w291) -> (w294:string[])
        n177 = Build Array(w290) -> (w293:string[])
        n178 = case shown="\"Stage\", Default" w278 {
          tunnel: w295 -> [w309 _]
          tunnel: w294 -> [w308 _]
          tunnel: w293 -> [w307 _]
          tunnel: w288 -> [w306 _]
          tunnel: w287 -> [w305 _]
          tunnel: w286 -> [w304 _]
          tunnel: w285 -> [w303 _]
          tunnel: w284 -> [w302 _]
          tunnel: w283 -> [w301 _]
          tunnel: [w300 w357] -> w282
          tunnel: w276 -> [w299 w358]
          tunnel: ctlSeqFNs_PI_SysNr."E710" ("DeviceNr.") -> [w298 _]
          tunnel: [w297 w355] -> w279
          tunnel: ctlSeqFNs_PI_SysNr."E517" ("DeviceNr.") -> [_ w355]
          tunnel: w275 -> [w296 _]
          frame "Stage", Default {
            n179 = stacked-sequence {
              seq-local: [w323 _ _ _] -> [_ w333 _ _]
              seq-local: [_ w338 _ _] -> [_ _ w343 _]
              seq-local: [_ _ w342 _] -> [_ _ _ w352]
              tunnel: w298 -> [w311 w341 w351 _]
              tunnel: w308 -> [_ w339 _ _]
              tunnel: w309 -> [w328 _ _ _]
              tunnel: w301 -> [w325 w332 w346 _]
              tunnel: w302 -> [w327 _ _ _]
              tunnel: w307 -> [w317 _ w350 _]
              tunnel: w304 -> [_ _ w344 _]
              tunnel: w303 -> [_ w334 _ _]
              tunnel: [_ _ _ w352] -> w300
              tunnel: w306 -> [w322 _ _ _]
              tunnel: w305 -> [w321 _ _ _]
              tunnel: w299 -> [w320 _ _ _]
              tunnel: [w311 _ _ _] -> w297
              tunnel: w296 -> [w316 _ _ _]
              frame #0 {
                n180 = Build Array(w325, w325) -> (w331:dbl[])
                n181 = Build Array(w316) -> (w315:dbl[])
                n182 = Build Array(w327) -> (w326:dbl[])
                n183 = call "WMS.vi"("System no."=w311, "Axes to set"=w328, "Wave storage max."=w331, "error in"=w320) -> ("error out"=w329:errorcluster)  [unwired: 1 in, 14 out]
                n184 = call "SPA_Hex.vi"("System no."=w311, "Designator to set"=w317, "Parameter value"=w326, "error in"=w329, "Parameter number (hex)"=u32[] [318767107]) -> ("error out"=w314:errorcluster)  [unwired: 1 in, 13 out]
                n185 = call "CCL.vi"("System no."=w311, "Command level"=1, "Password"="ADVANCED", "error in"=w314) -> ("error out"=w310:errorcluster)  [unwired: 14 in, 1 out]
                n186 = call "SPA_Hex.vi"("System no."=w311, "Designator to set"=w317, "Parameter value"=w315, "error in"=w310, "Parameter number (hex)"=u32[] [318767369]) -> ("error out"=w319:errorcluster)  [unwired: 1 in, 13 out]
                n187 = call "TWS.vi"("System no."=w311, "Wavepoint"=w322, "Trigger value"=w321, "error in"=w319) -> ("error out"=w323:errorcluster)  [unwired: 1 in, 14 out]
                "Writing" <- TRUE
              }
              frame #1 {
                w335 = u16 6 items=["SIN", "POL", "TAN", "PNT", "SIN_P", "LIN", "RAMP"] ("Waveform")
                w336 = 0.0 ("J")
                # "CJAO"
                n188 = Bundle("Points"=w332, "J"=w336, "X length"=w334, "J"=w336) -> (w337:T6)  [unwired: 1 out]
                n189 = call "WAV.vi"("System no."=w341, "Waveform"=w335, "Affected axes"=w339, "Append? (&)"=FALSE, "error in"=w333, "N"=w332, "Segment length"=w332, "RAMP Parameters"=w337) -> ("error out"=w338:errorcluster)  [unwired: 10 in, 9 out]
              }
              frame #2 {
                w348 = u16 5 items=["SIN", "POL", "TAN", "PNT", "SIN_P", "LIN", "RAMP"] ("Waveform")
                w345 = 0.0 ("J")
                # "Y axis: step upwards"
                # "X0 = N  --> Step at the\nend of the period."
                # "JAO"
                n190 = Bundle("J"=w345, "Stepsize Y"=w344, "J"=w345) -> (w349:cluster{"J":dbl, "Stepsize Y ":dbl, "J":dbl})  [unwired: 1 out]
                n191 = call "WAV.vi"("System no."=w351, "Waveform"=w348, "Affected axes"=w350, "Append? (&)"=FALSE, "error in"=w343, "Xo"=w346, "N"=w346, "Segment length"=w346, "LIN Parameters"=w349) -> ("error out"=w342:errorcluster)  [unwired: 9 in, 9 out]
              }
              frame #3 {
                n192 = local write "Writing"(FALSE) -> ()
              }
            }
          }
          frame "Mirror" {
            w380 = 1000  # N
            w356 = i32[] [1]  # Wavegenerator table rate
            w366 = 1000  # Segment length
            w354 = 50
            w377 = i32[] [1] ("Generator ID")
            w359 = string[] ["1"] ("Affected axes")
            w381 = u16 4 items=["SIN", "POL", "TAN", "PNT", "SIN_P", "LIN", "RAMP"] ("Waveform")
            # "Trigger"
            # "Setup trigger"
            # "Setup wavegen"
            # "Define sine wave"
            # "Generate trigger points"
            n193 = To Double Precision Float(number=w354) -> (double precision float=w364:dbl)
            n194 = To Double Precision Float(number=w366) -> (double precision float=w365:dbl)
            n195 = Divide(x=w365, y=w364) -> (x/y=w363:dbl)
            n196 = To Long Integer(number=w363) -> (32bit integer=w362:i32)
            n197 = for {
              N: w354 -> [_]
              tunnel: [w386] -> w369 mode=indexing
              tunnel: [w386] -> w370 mode=indexing
              tunnel: w362 -> [w383]
              tunnel: [w384] -> w367 mode=indexing
              i -> [w382]
              w386 = 1 ("N 2")
              n198 = Multiply(x=w382, y=w383) -> (x*y=w385:i32)
              n199 = Increment(x=w385) -> (x+1=w384:i32)
            }
            n200 = call "WAV.vi"("System no."=w355, "Waveform"=w381, "Affected axes"=w359, "error in"=w358, "Xo"=0, "N"=w380, "Segment length"=w366, "SIN_P Parameters"=cluster{"C":dbl, "A":dbl, "O":dbl} {"C"=500.0, "A"=20.0, "O"=0.0}) -> ("error out"=w360:errorcluster)  [unwired: 10 in, 9 out]
            n201 = call "WTR.vi"("System no."=w355, "Generator ID"=w377, "Table rate"=w356, "Interpolation type"=i32[] [0], "error in"=w360) -> ("error out"=w378:errorcluster)  [unwired: 14 out]
            n202 = call "WGC.vi"("System no."=w355, "Affected axes"=w359, "Cycles"=w377, "error in"=w378) -> ("error out"=w376:errorcluster)  [unwired: 15 out]
            n203 = call "TWC.vi"("System no."=w355, "error in"=w376) -> ("error out"=w375:errorcluster)  [unwired: 17 out]
            n204 = call "CTO.vi"("System no."=w355, "TriggerOut to set"=string[] ["1"] ("DIO-Line for TriggerOut"), "error in"=w375, "CTO parameter ID"=i32[] [3], "Parameter value"=string[] ["4"]) -> ("error out"=w374:errorcluster)  [unwired: 1 in, 13 out]
            n205 = call "TWS.vi"("System no."=w355, "Wavepoint"=w367, "Trigger value"=w370, "Switch"=w369, "error in"=w374) -> ("error out"=w357:errorcluster)  [unwired: 14 out]
          }
        }
        n206 = call "ERR?.vi"("System no."=w279, "error in"=w282) -> ("error out"=w292:errorcluster)  [unwired: 17 out]
        n207 = call "GCSTranslateError.vi"("error in"=w292) -> ("error out"=w281:errorcluster)  [unwired: 18 out]
      }
      event "Set Temp": Value Change {
        n208 = event-data() -> ()  [unwired: 1 in, 6 out]
        n209 = call "Prompt User for Input"("error in (no error)"=w400) -> ("Temperature"=w398:dbl, "error out"=w399:errorcluster)  [unwired: 16 in, 1 out]
        n210 = call "CheckTemperature.vi"("error in (no error)"=w399, "temperature in"=w398) -> ()  [unwired: 8 in, 2 out]
      }
      event "AOTF Settings": Value Change {
        n211 = event-data() -> ()  [unwired: 1 in, 6 out]
        n212 = stacked-sequence {
          seq-local: [w460 _ _] -> [_ w471 _]
          seq-local: [_ w472 _] -> [_ _ w491]
          tunnel: [w469 _ _] -> w430
          tunnel: [w468 _ _] -> w429
          tunnel: [w467 _ _] -> w428
          tunnel: [w466 _ _] -> w427
          tunnel: [w465 _ _] -> w426
          tunnel: [w464 _ _] -> w425
          tunnel: [w463 _ _] -> w424
          tunnel: [w462 _ _] -> w423
          tunnel: w422 -> [w461 _ _]
          tunnel: [_ w480 _] -> w421
          tunnel: [_ w479 _] -> w420
          tunnel: [_ w478 _] -> w419
          tunnel: [_ w477 _] -> w418
          tunnel: [_ w476 _] -> w417
          tunnel: [_ w475 _] -> w416
          tunnel: [_ w474 _] -> w415
          tunnel: [_ w473 _] -> w414
          tunnel: [_ _ w490] -> w409
          tunnel: [_ _ w488] -> w413
          tunnel: [_ _ w487] -> w412
          tunnel: [_ _ w486] -> w411
          tunnel: [_ _ w485] -> w410
          tunnel: [_ _ w484] -> w408
          tunnel: [_ _ w489] -> w407
          tunnel: [_ _ w483] -> w406
          tunnel: [_ _ w482] -> w405
          tunnel: [_ w470 _] -> w404
          tunnel: [w459 _ _] -> w403
          tunnel: [_ _ w481] -> w402
          frame #0 {
            n213 = call "Define ON/OFF State of AOTF Channels"("error in (no error)"=w461) -> ("Channel 8 On/Off"=w462:bool, "Channel 7 On/Off"=w463:bool, "Channel 6 On/Off"=w464:bool, "Channel 5 On/Off"=w465:bool, "Channel 4 On/Off"=w466:bool, "Channel 3 On/Off"=w467:bool, "Channel 2 On/Off"=w468:bool, "Channel 1 On/Off"=w469:bool, "OK"=w459:bool, "error out"=w460:errorcluster)  [unwired: 9 in]
          }
          frame #1 {
            n214 = call "Define power intensity of AOTF Channels"("error in (no error)"=w471) -> ("Channel 8 Power"=w473:dbl, "Channel 7 Power"=w474:dbl, "Channel 6 Power"=w475:dbl, "Channel 5 Power"=w476:dbl, "Channel 4 Power"=w477:dbl, "Channel 3 Power"=w478:dbl, "Channel 2 Power"=w479:dbl, "Channel 1 Power"=w480:dbl, "OK"=w470:bool, "error out"=w472:errorcluster)  [unwired: 9 in]
          }
          frame #2 {
            n215 = call "Define wavelength of AOTF Channels"("error in (no error)"=w491) -> ("Wavelength Channel 8"=w490:dbl, "Wavelength Channel 7"=w488:dbl, "Wavelength Channel 6"=w487:dbl, "Wavelength Channel 5"=w483:dbl, "Wavelength Channel 4"=w486:dbl, "Wavelength Channel 3"=w485:dbl, "Wavelength Channel 2"=w484:dbl, "Wavelength Channel 1"=w489:dbl, "OK"=w481:bool, "error out"=w482:errorcluster)  [unwired: 9 in]
          }
        }
        n216 = Compound Arithmetic op=AND(w404, w403, w402) -> (w401:bool)
        n217 = case shown="True" w401 {
          tunnel: [w432 w458] -> w431
          tunnel: w430 -> [_ w457]
          tunnel: w429 -> [_ w456]
          tunnel: w428 -> [_ w455]
          tunnel: w427 -> [_ w454]
          tunnel: w426 -> [_ w453]
          tunnel: w425 -> [_ w452]
          tunnel: w424 -> [_ w451]
          tunnel: w423 -> [_ w450]
          tunnel: w421 -> [_ w449]
          tunnel: w420 -> [_ w448]
          tunnel: w419 -> [_ w447]
          tunnel: w418 -> [_ w446]
          tunnel: w417 -> [_ w445]
          tunnel: w416 -> [_ w444]
          tunnel: w415 -> [_ w443]
          tunnel: w414 -> [_ w442]
          tunnel: w413 -> [_ w441]
          tunnel: w412 -> [_ w440]
          tunnel: w411 -> [_ w439]
          tunnel: w410 -> [_ w438]
          tunnel: w409 -> [_ w437]
          tunnel: w408 -> [_ w436]
          tunnel: w407 -> [_ w435]
          tunnel: w406 -> [_ w434]
          tunnel: w405 -> [w432 w433]
          frame False {
          }
          frame True {
            n218 = call "UpdateLaserAOTFSettings.vi"("3.LaserChannel ON/OFF"=w455, "4.LaserChannel ON/OFF"=w454, "On/OFF  Power 2"=w453, "6.LaserChannel ON/OFF"=w452, "7.LaserChannel ON/OFF"=w451, "8.LaserChannel ON/OFF"=w450, "1.Laser Channel Power / [%]"=w449, "2.Laser Channel Power / [%]"=w448, "2.LaserChannel ON/OFF"=w456, "3.Laser Channel Power / [%]"=w447, "On/OFF  Power"=w457, "4.Laser Channel Power / [%]"=w446, "5.Laser Channel Power / [%]"=w445, "error in"=w433, "6.Laser Channel Power / [%]"=w444, "7.Laser Channel Power / [%]"=w443, "8.Laser Channel Power / [%]"=w442, "1.Laser Channel Wavelength 8"=w437, "1.Laser Channel Wavelength 7"=w441, "1.Laser Channel Wavelength 6"=w440, "Wavelength 2"=w434, "1.Laser Channel Wavelength 4"=w439, "1.Laser Channel Wavelength 3"=w438, "1.Laser Channel Wavelength 2"=w436, "Wavelength"=w435) -> ("error out"=w458:errorcluster)  [unwired: 2 in]
          }
        }
      }
      event "Get Beam Diagnostic": Value Change {
        n219 = event-data() -> ()  [unwired: 1 in, 6 out]
        n220 = global write "GlobalGetBeamDiagnostics.vi" "Get Beam Diagnostic"("Get Beam Diagnostic") -> ()
      }
      event "Stop Beam Diagnostic": Value Change {
        n221 = event-data() -> ()  [unwired: 1 in, 6 out]
        n222 = global write "GlobalStopGetBeamDiagnostics.vi" "Stop Beam Diagnostic"("Stop Beam Diagnostic") -> ()
      }
      event "Laser Power": Value Change {
        n223 = event-data() -> ()  [unwired: 1 in, 6 out]
        n224 = call "LaserStartUpSequence.vi"("error in (no error)"=w494) -> ("error out"=w495:errorcluster)  [unwired: 10 in]
      }
      event "Camera Settings": Value Change {
        n225 = event-data() -> ()  [unwired: 1 in, 6 out]
        n226 = call "Camera GAIN"("error in (no error)"=w497) -> ("Gain"=w498:dbl, "error out"=w496:errorcluster)  [unwired: 16 in, 1 out]
        n227 = global write "GlobalSetGetConfigureCamera.vi" "gain"(w498) -> ()
      }
      event "Brightness::Value": Value Change {
        n228 = event-data() -> ()  [unwired: 1 in, 6 out]
        n229 = property on="Brightness::Value" class="DigNum (strict)"("Value"="Brightness::Value") -> ()  [unwired: 2 in, 2 out]
      }
      event "Gain::Value": Value Change {
        n230 = event-data() -> ()  [unwired: 1 in, 6 out]
        n231 = property on="Gain::Value" class="DigNum (strict)"("Value"="Gain::Value") -> ()  [unwired: 2 in, 2 out]
      }
      event "Emergency Exit": Value Change {
        n232 = event-data() -> ()  [unwired: 1 in, 6 out]
        n233 = stacked-sequence {
          seq-local: [w510 _ _] -> [_ w513 _]
          seq-local: [_ w512 _] -> [_ _ w519]
          tunnel: "Emergency Exit" -> [w511 _ _]
          tunnel: [w511 _ _] -> w501
          tunnel: w506 -> [w510 _ _]
          tunnel: [_ _ w518] -> w505
          frame #0 {
            n234 = global write "GlobalStopGetBeamDiagnostics.vi" "Stop Beam Diagnostic"(w511) -> ()
            n235 = global write "GlobalExitVar.vi" "Emergency Exit"(w511) -> ()
          }
          frame #1 {
            n236 = Concatenate Strings("daughter disable" ("string"), "\r") -> (w516:string)
            n237 = call "CTI_AOTF.vi"("error in"=w513, "String"=w516, "VISA resource name 2"=refnum<visa-resource-name> "USB0::0x16C7::0x0001::NI-VISA-20001::RAW") -> ("error out"=w512:errorcluster)  [unwired: 7 in, 1 out]
          }
          frame #2 {
            n238 = case shown="No Error" w519 {
              selector: w519 -> [w531 w536]
              tunnel: refnum<visa-resource-name> "COM3" ("VISA resource name in") -> [w532 w535]
              tunnel: [w531 w534] -> w525
              tunnel: [w532 w533] -> w524
              frame No Error {
              }
              frame Error {
                n239 = VISA Close(VISA resource name=w535, error in (no error)=w536) -> (error out=w537:errorcluster)
                n240 = call "Koheras_Init.vi"("error in"=w537, "VISA resource name"=w535) -> ("error out"=w534:errorcluster, "VISA resource name out"=w533:refnum<visa-resource-name>)  [unwired: 8 in]
              }
            }
            n241 = Number To Decimal String(number=0 ("laserPower"), width (-)=i16 0) -> (decimal integer string=w530:string)
            n242 = Concatenate Strings("set power " ("string"), w530) -> (w528:string)
            n243 = Build Array(w528) -> (w521:string[])
            n244 = Build Array(9 ("new element/subarray")) -> (w520:i32[])
            n245 = call "Koheras_get_set_Status.vi"("error in"=w525, "Array 2"=w520, "Array"=w521, "VISA resource name in"=w524) -> ("error out"=w518:errorcluster)  [unwired: 5 in, 2 out]
          }
        }
        n246 = while {
          shift-right: [w538] -> w504
          shift-left: w505 -> [w542]
          stop <- w539 stop-if-true
          n247 = Wait Until Next ms Multiple(millisecond multiple=u32 1000) -> ()  [unwired: 1 out]
          n248 = call "CheckTemperature.vi"("error in (no error)"=w542, "temperature in"=10) -> ("error out"=w538:errorcluster, "TemperatureReached"=w539:bool)  [unwired: 8 in]
        }
        n249 = call "ShutDown.vi"("error in (no error)"=w504) -> ("error out"=w503:errorcluster)  [unwired: 1 in, 1 out]
        n250 = flat-sequence {
          tunnel: w503 -> [w509]
          tunnel: [w509] -> w502
          tunnel: w501 -> [w508]
          frame #0 {
            n251 = Quit LabVIEW(quit? (T)=w508) -> ()
          }
        }
      }
    }
  }
